vi "Date.vi"(8 "error in":errorcluster, 11 "Refnum in":refnum<k34>) -> (0 "error out":errorcluster, 3 "Refnum out":refnum<k34>)   [LabVIEW 2019]
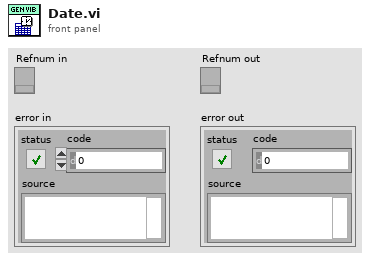
[diagram p1: front panel]
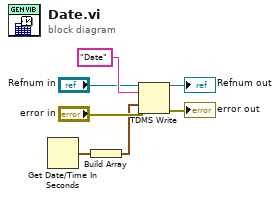
[diagram p0: block diagram]
diagram:
  n1 = Get Date/Time In Seconds() -> (seconds since 1Jan1904=w5:timestamp)
  n2 = Build Array(w5) -> (w4:timestamp[])
  n3 = TDMS Write(0:"Refnum in", 5:"Date" ("group name in (Untitled)"), 9:w4, 11:"error in") -> (4:→"Refnum out":refnum<k34>, 15:→"error out":errorcluster)  [unwired: 2 in, 2 out]
